vi "RANDOMTOBALLRACK.vi"   [LabVIEW 2016, in "Test2.lvrbt"]
uses:
  Test2.lvrbt
  <vilib>/NXT/Block Support/NXT_InputPort.ctl
  <vilib>/NXT/Hardware/Plugins/Tetrix DC Motor/TetrixDCMotorAddress.ctl
  <vilib>/NXT/NXTIO Xnodes/NXTIONodeSubVIs/TETRIX IO Move DC Motors.vi
  <vilib>/NXT/Dual Mode Library/Waits/Wait_EV3_Ultrasonic_Centimeter_Closer.vi
  <vilib>/NXT/NXTIO Xnodes/NXTIONodeSubVIs/TETRIX IO Stop DC Motors.vi
  <vilib>/NXT/Dual Mode Library/Waits/Wait_Num.vi
  <vilib>/NXT/Dual Mode Library/Waits/Wait_Touch.vi
  <vilib>/NXT/Subs/LVHSConnector.ctl
  <vilib>/NXT/NXTIO Xnodes/AddressXNode/NXTIOAddress.xnode
  <vilib>/NXT/NXTIO Xnodes/NXTIOXNode/NXTIO.xnode
  <vilib>/NXT/LegoClasses/BrickReference/BrickReference.lvclass
types:
  T1 = typedef "NXT_InputPort.ctl" = u32
  T2 = typedef "TetrixDCMotorAddress.ctl" = i32
  T3 = typedef "LVHSConnector.ctl" = refnum<class "BrickReference.lvclass">
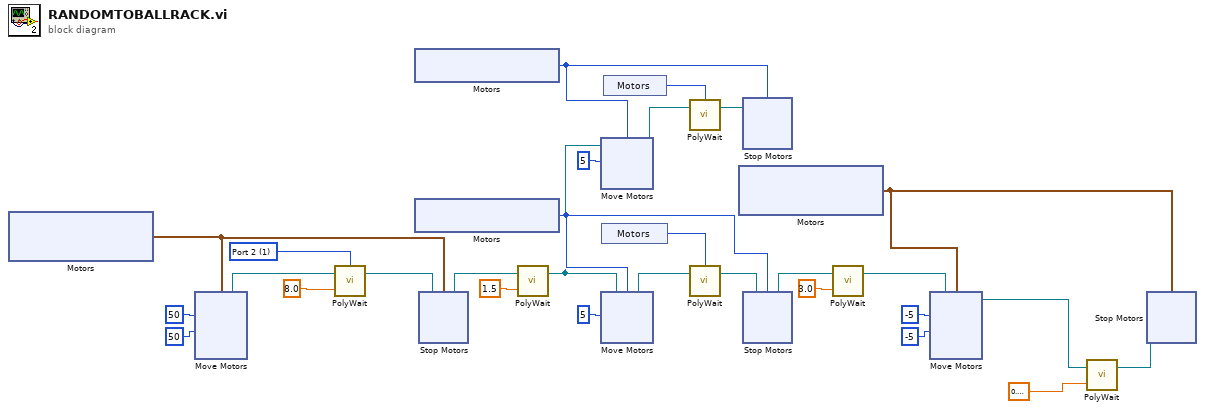
[diagram p0: block diagram]
diagram:
  w10 = T1 1 items=["Port 1", "Port 2", "Port 3", "Port 4"] ("Port (Port 1)")
  n1 = xnode "Motors"() -> ("Motor"=w24:cluster{"TetrixDCMotor":T2, "TetrixDCMotor":T2})
  n2 = xnode "Move Motors"("Power/Speed 2"=i8 50, "Power/Speed 1"=i8 50, "Motors"=w24) -> ("NXT/EV3"=w27:T3)  [unwired: 1 in]
  n3 = call-poly <vilib>:"PolyWait.vi"("Centimeters (40)"=sgl 8.0, "NXT/EV3"=w27, "Port (Port 1)"=w10) -> ("NXT/EV3"=w25:T3)  [unwired: 1 in]
  n4 = xnode "Motors"() -> ("Motor"=w20:T2)
  n5 = xnode "Motors"() -> ("Motor"=w15:T2)
  n6 = xnode "Stop Motors"("Motors"=w24, "NXT/EV3"=w25) -> ("NXT/EV3"=w18:T3)
  n7 = call-poly <vilib>:"PolyWait.vi"("Time (1 sec)"=sgl 1.5, "NXT/EV3"=w18) -> ("NXT/EV3"=w13:T3)  [unwired: 2 in]
  n8 = xnode "Move Motors"("Power/Speed 1"=i8 5, "Motors"=w20, "NXT/EV3"=w13) -> ("NXT/EV3"=w22:T3)
  n9 = xnode "Move Motors"("Power/Speed 1"=i8 5, "Motors"=w15, "NXT/EV3"=w13) -> ("NXT/EV3"=w16:T3)
  n10 = xnode "Motors"() -> ("Sensor"=w12:T1)
  n11 = xnode "Motors"() -> ("Sensor"=w11:T1)
  n12 = call-poly <vilib>:"PolyWait.vi"("NXT/EV3"=w22, "Port (Port 1)"=w11) -> ("NXT/EV3"=w21:T3)  [unwired: 2 in]
  n13 = call-poly <vilib>:"PolyWait.vi"("NXT/EV3"=w16, "Port (Port 1)"=w12) -> ("NXT/EV3"=w14:T3)  [unwired: 2 in]
  n14 = xnode "Motors"() -> ("Motor"=w7:cluster{"TetrixDCMotor":T2, "TetrixDCMotor":T2})
  n15 = xnode "Stop Motors"("Motors"=w20, "NXT/EV3"=w21) -> ()  [unwired: 1 out]
  n16 = xnode "Stop Motors"("Motors"=w15, "NXT/EV3"=w14) -> ("NXT/EV3"=w9:T3)
  n17 = call-poly <vilib>:"PolyWait.vi"("Time (1 sec)"=sgl 3.0, "NXT/EV3"=w9) -> ("NXT/EV3"=w5:T3)  [unwired: 2 in]
  n18 = xnode "Move Motors"("Power/Speed 2"=i8 -5, "Power/Speed 1"=i8 -5, "Motors"=w7, "NXT/EV3"=w5) -> ("NXT/EV3"=w2:T3)
  n19 = call-poly <vilib>:"PolyWait.vi"("Time (1 sec)"=sgl 0.2, "NXT/EV3"=w2) -> ("NXT/EV3"=w1:T3)  [unwired: 2 in]
  n20 = xnode "Stop Motors"("Motors"=w7, "NXT/EV3"=w1) -> ()  [unwired: 1 out]
